vi "Coord window-Save setup.vi"(8 "error in (no error)":errorcluster) -> (0 "error out":errorcluster)   [LabVIEW 2013]
uses:
  Visualisation/Functional Imaging Viewer/Typedefs/Get-Set-Clear Control.ctl
  Globals/Coord window-Globals.vi
  Typedefs/Save-Load enum.ctl
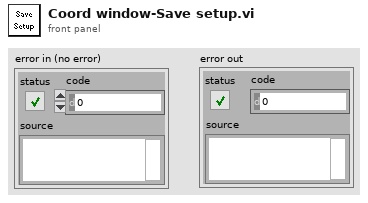
[diagram p1: front panel]
types:
  T1 = typedef "Coordinate list window refs.ctl" = cluster{"Window Name (i.e. Key)":string, "menu reference":refnum<k9>, "VI's reference":refnum<vi>, "Pane 1":refnum<vi>, "Pane 2":refnum<vi>, "Coord Listbox":refnum<vi>, "File name":refnum<vi>, "Picture Map":refnum<vi>, "Stage XYZ Position ind.":refnum<vi>}
  T2 = typedef "Get-Set-Clear Control.ctl" = enum16{"Get", "Set", "Clear"}
  T3 = typedef "Save-Load enum.ctl" = enum16{"Save to file", "Load from file", "Compare from file"}
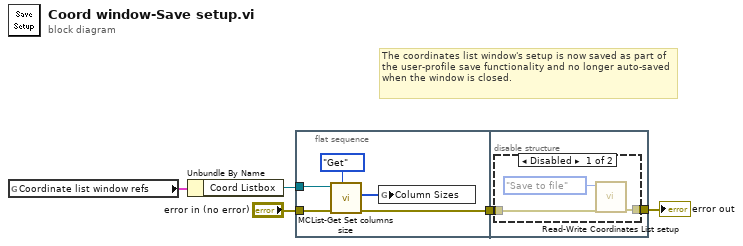
[diagram p0: block diagram]
diagram:
  # "The coordinates list window's setup is now saved as part of the user-profile save functionality and no longer auto-saved when the window is closed."
  n1 = global read "Coord window-Globals.vi" "Coordinate list window refs"() -> (w2:T1)
  n2 = Unbundle By Name(w2) -> ("Coord Listbox"=w3:refnum<vi>)
  n3 = flat-sequence {
    tunnel: [w8] -> w5
    tunnel: "error in (no error)" -> [w7]
    tunnel: w3 -> [w6]
    tunnel: w5 -> [w12]
    tunnel: [w11] -> w4
    frame #0 {
      n4 = call "MCList-Get Set columns size.vi"("Function"=Get-Set-Clear_Control."Get", "error in (no error)"=w7, "Listbox ref"=w6) -> ("Error out"=w8:errorcluster, "Sizes"=w9:u32[])  [unwired: 7 in]
      n5 = global write "Coord window-Globals.vi" "Column Sizes"(w9) -> ()
    }
    frame #1 {
      n6 = disable-structure shown="Disabled" {
        disable-tunnel: w12 -> [w15 w16]
        disable-tunnel: [w14 w16] -> w11
        frame Disabled {
          n7 = call "Read-Write Coordinates List setup.vi"("error in"=w15, "Function"=Save-Load_enum."Save to file") -> ("error out"=w14:errorcluster)  [unwired: 9 in]
        }
        frame Enabled {
        }
      }
    }
  }
  "error out" <- w4
